vi "AppleScript Main.vi"() -> ()   [LabVIEW 2017, in "Apple script.lvlib"]
doc: "Main block for AppleScript.\nPut this in the autonomous vi. Do not place this inside of a loop."
uses:
  Apple script.lvlib
  Robot Global Data.vi
  <vilib>/Rock Robotics/Network Tables/NT Read Number.vi
  <vilib>/Rock Robotics/Network Tables/NT Read String.vi
panel:
  out "Loop 1":u32
  # "AppleScript\nAutonomous Scripting Language for LabVIEW\nCreated by Cory Lynch\nFRC Team 2067"
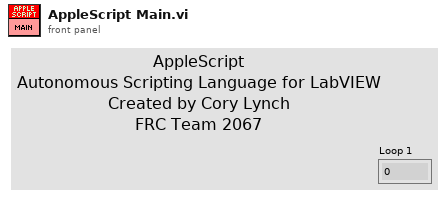
[diagram p1: front panel]
types:
  T1 = cluster{"If Index":i16, "If Boolean":bool, "Execute Index":i16, "Execute Boolean":bool, "Group Index":i16[], "Group Boolean":bool[]}[]
  T2 = cluster{"If Index":i32, "If Boolean":bool, "Execute Index":i32, "Execute Boolean":bool, "Group Index":i32[], "Group Boolean":bool[]}[]
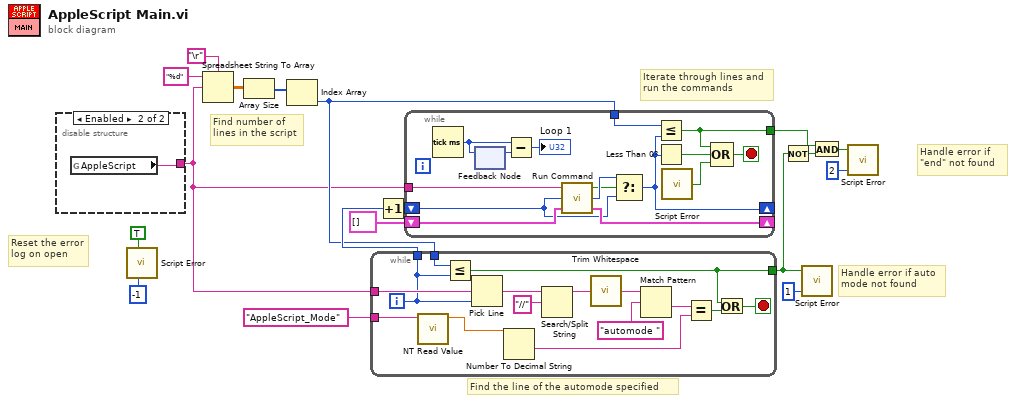
[diagram p0: block diagram]
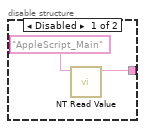
[diagram p2: hidden frame]
diagram:
  # "Find number of \nlines in the script"
  # "Handle error if\n\"end\" not found"
  # "Handle error if auto\nmode not found"
  # "Iterate through lines and\nrun the commands"
  # "Find the line of the automode specified"
  # "Reset the error\nlog on open"
  n1 = disable-structure shown="Enabled" {
    disable-tunnel: [w20 w21] -> w1
    frame Disabled {
      n2 = call-poly <vilib>:"NT Read Value.vi"("Name"="AppleScript_Main") -> ("String"=w20:string)  [unwired: 9 in, 1 out]
    }
    frame Enabled {
      n3 = global read "Robot Global Data.vi" "AppleScript"() -> (w21:string)
    }
  }
  n4 = call "Script Error.vi"("Reset Log"=TRUE, "Line Number"=-1) -> ()  [unwired: 3 in, 1 out]
  n5 = Spreadsheet String To Array(delimiter (Tab)="\r", format string="%d", spreadsheet string=w1) -> (array=w17:dbl[][])  [unwired: 1 in]
  n6 = Array Size(array=w17) -> (size(s)=w14:i32[])
  n7 = Index Array(array=w14) -> (element=w8:i32)  [unwired: 1 in]
  n8 = while {
    tunnel: w1 -> [w30]
    tunnel: [w26] -> w18
    tunnel: w8 -> [w27]
    tunnel: [w24] -> w7
    tunnel: "AppleScript_Mode" ("Name") -> [w23]
    i -> [w26]
    stop <- w25 stop-if-true
    n9 = call-poly <vilib>:"NT Read Value.vi"("Name"=w23) -> ("Numeric"=w22:dbl)  [unwired: 9 in, 1 out]
    n10 = Less Or Equal?(x=w27, y=w26) -> (x <= y?=w24:bool)
    n11 = Pick Line(multi-line string=w30, line index=w26) -> (output string=w29:string)  [unwired: 1 in]
    n12 = Number To Decimal String(number=w22) -> (decimal integer string=w34:string)  [unwired: 1 in]
    n13 = Search/Split String(string=w29, search string/char (-)="//") -> (substring before match=w32:string)  [unwired: 1 in, 2 out]
    n14 = call <vilib>:"Trim Whitespace.vi"("string"=w32) -> ("trimmed string"=w31:string)  [unwired: 1 in]
    n15 = Match Pattern(string=w31, regular expression="automode ") -> (after substring=w35:string)  [unwired: 1 in, 3 out]
    n16 = Equal?(x=w35, y=w34) -> (x = y?=w28:bool)
    n17 = Or(x=w24, y=w28) -> (x .or. y?=w25:bool)
  }
  n18 = Increment(x=w18) -> (x+1=w5:i32)
  n19 = while {
    tunnel: w1 -> [w45]
    shift-right: [w51] -> _
    shift-left: w5 -> [w40]
    tunnel: w8 -> [w50]
    tunnel: [w49] -> w11
    shift-right: [w42] -> _
    shift-left: T1 [] ("Values") -> [w41]
    stop <- w47 stop-if-true
    n20 = Tick Count (ms)() -> (millisecond timer value=w38:u32)
    n21 = feedback #1() -> (w39:u32)  [unwired: 1 in]
    n22 = feedback-in #1(w38) -> ()
    n23 = Subtract(x=w38, y=w39) -> (x-y=→"Loop 1":u32)
    n24 = call "Run Command.vi"("Values"=w41, "Line Index In"=w40, "Script"=w45) -> ("Values out"=w42:T2, "Line Index Out"=w44:i32, "Done"=w43:bool)
    n25 = Select(t=w44, s=w43, f=w40) -> (s? t:f=w51:i32)
    n26 = Less Or Equal?(x=w50, y=w51) -> (x <= y?=w49:bool)
    n27 = Less Than 0?(x=w51) -> (x < 0?=w48:bool)
    n28 = call "Script Error.vi"() -> ("Error?"=w46:bool)  [unwired: 5 in]
    n29 = Compound Arithmetic op=OR(w49, w48, w46) -> (w47:bool)
  }
  n30 = Not(x=w7) -> (.not. x?=w10:bool)
  n31 = call "Script Error.vi"("Error?"=w7, "Error Code"=1) -> ()  [unwired: 3 in, 1 out]
  n32 = And(x=w11, y=w10) -> (x .and. y?=w9:bool)
  n33 = call "Script Error.vi"("Error?"=w9, "Error Code"=2) -> ()  [unwired: 3 in, 1 out]
